vi "SERIAL_WRITE_INT_TO_STRING.vi"(0 "buffer in":string, 5 "ENVIAR":bool, 7 "bomba on/off":i32, 9 "tiempo":i32, 11 "fin de cadena":string=" S") -> (4 "buffer out":string, 6 "int to string out":string, 10 "dato a enviar":string, 15 "ok":bool)   [LabVIEW 2017]
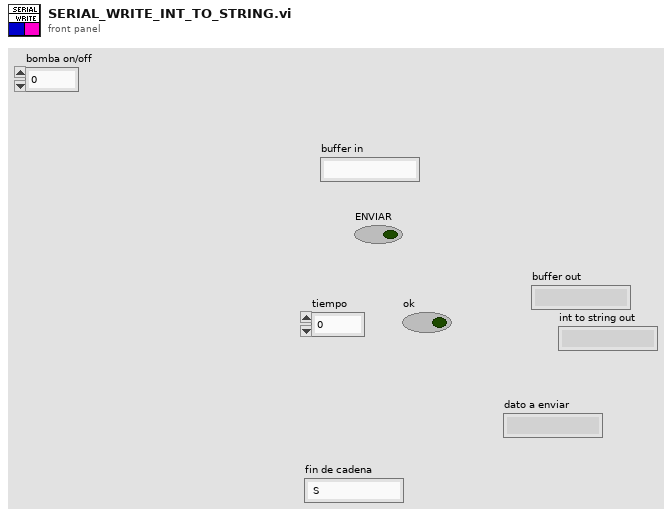
[diagram p1: front panel]
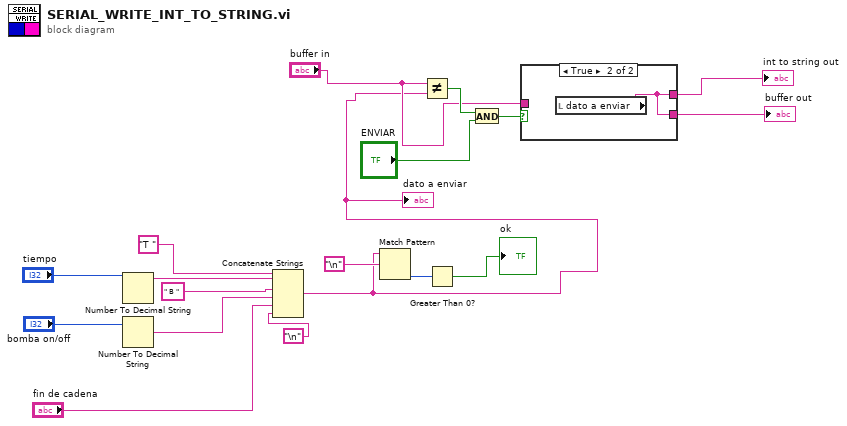
[diagram p0: block diagram]
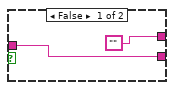
[diagram p2: hidden frame]
diagram:
  n1 = Number To Decimal String(number="tiempo") -> (decimal integer string=w9:string)  [unwired: 1 in]
  n2 = Number To Decimal String(number="bomba on/off") -> (decimal integer string=w1:string)  [unwired: 1 in]
  n3 = Concatenate Strings("T " ("string"), w9, " B " ("string"), w1, "fin de cadena", "\n") -> (w6:string)
  "dato a enviar" <- w6
  n4 = Match Pattern(string=w6, regular expression="\n") -> (offset past match=w11:i32)  [unwired: 1 in, 3 out]
  n5 = Not Equal?(x="buffer in", y=w6) -> (x != y?=w17:bool)
  n6 = Greater Than 0?(x=w11) -> (x > 0?=→"ok":bool)
  n7 = And(x=w17, y="ENVIAR") -> (x .and. y?=w18:bool)
  n8 = case shown="True" w18 {
    tunnel: ["" w21] -> w13
    tunnel: [w19 w21] -> w14
    tunnel: "buffer in" -> [w19 _]
    frame False {
    }
    frame True {
      n9 = local read "dato a enviar"() -> (w21:string)
    }
  }
  "buffer out" <- w14
  "int to string out" <- w13
